vi "DO Read Port.vi"(8 "error in (no error)":errorcluster caption="错误输入（无错误）", 9 "Value":u32, 10 "Port":u16, 11 "CardNumber":u16) -> (0 "error out":errorcluster caption="错误输出", 1 "Value out":u32, 3 "function return":i16)   [LabVIEW 2017, in "Adlink IO.lvlib"]
doc: "I16 __stdcall DO_ReadPort(U16 CardNumber, U16 Port, U32 *Value);"
uses:
  Adlink IO.lvlib
  PCI-Dask.dll
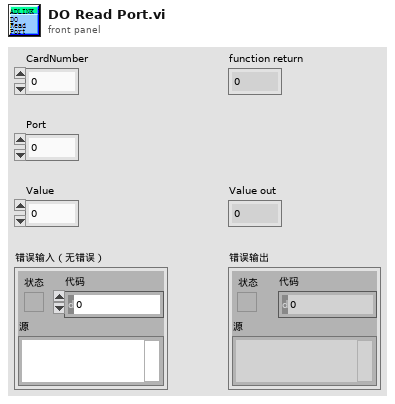
[diagram p1: front panel]
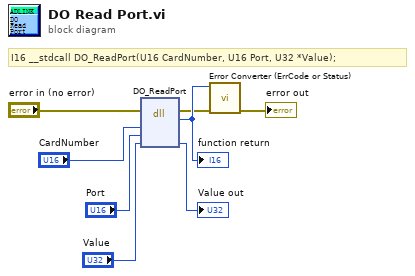
[diagram p0: block diagram]
diagram:
  # "I16 __stdcall DO_ReadPort(U16 CardNumber, U16 Port, U32 *Value);"
  n1 = dll-call lib="PCI-Dask.*" fn="DO_ReadPort"(error in="error in (no error)", "CardNumber"="CardNumber", "Port"="Port", "Value"="Value") -> (error out=w2:errorcluster, w8:i16, "Value"=→"Value out":u32)  [unwired: 4 in, 1 out]
  "function return" <- w8
  n2 = call "Error Converter (ErrCode or Status).vi"("error in (no error)"=w2, "error code"=w8) -> ("error out"=→"error out":errorcluster)  [unwired: 9 in]
